vi "ReleaseBuffer.vi"(8 "error in (no error)":errorcluster, 10 "Pointer and BufferSize":u64[](array[numeric])) -> (0 "error out":errorcluster)   [LabVIEW 2024]
uses:
  <vilib>/Utility/error.llb/DialogType.ctl
panel:
  in  "type of dialog (OK msg:1)":T1=4 items=["no dialog", "OK message", "continue or stop message", "OK message + warnings", "continue/stop + warnings"]
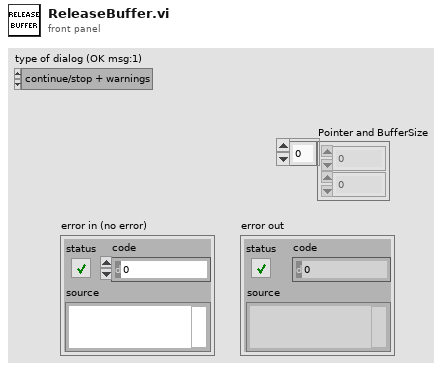
[diagram p1: front panel]
types:
  T1 = typedef "DialogType.ctl" = u16
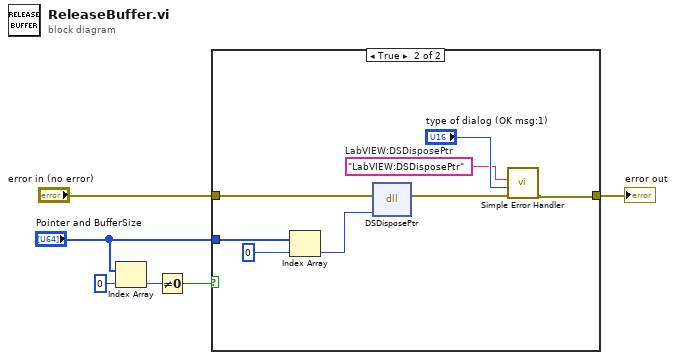
[diagram p0: block diagram]
diagram:
  n1 = Index Array(array="Pointer and BufferSize", index=0) -> (element=w2:u64)
  n2 = Not Equal To 0?(x=w2) -> (x != 0?=w1:bool)
  n3 = case shown="True" w1 {
    tunnel: [w7 w8] -> w6
    tunnel: "error in (no error)" -> [w7 w15]
    tunnel: "Pointer and BufferSize" -> [_ w12]
    frame False {
    }
    frame True {
      w10 = "LabVIEW:DSDisposePtr"  # LabVIEW:DSDisposePtr
      n4 = Index Array(array=w12, index=0) -> (element=w14:u64)
      n5 = dll-call lib="LabVIEW" fn="DSDisposePtr"(error in=w15, "Pointer"=w14) -> (error out=w9:errorcluster)  [unwired: 4 in, 1 out]
      n6 = call <vilib>:"Simple Error Handler.vi"("error source (\" \")"=w10, "type of dialog (OK msg:1)"="type of dialog (OK msg:1)", "error in (no error)"=w9) -> ("error out"=w8:errorcluster)  [unwired: 2 in, 4 out]
    }
  }
  "error out" <- w6
